vi "Search in 1D Array.vi"(2 "Task in":refnum<class "Task.lvclass">, 3 "Task Array":refnum<class "Task.lvclass">[](array[class])) -> (0 "index of element":i32, 1 "Task":refnum<class "Task.lvclass">)   [LabVIEW 2017, in "Task Interface.lvlib" / "Task.lvclass"]
uses:
  Task.lvclass
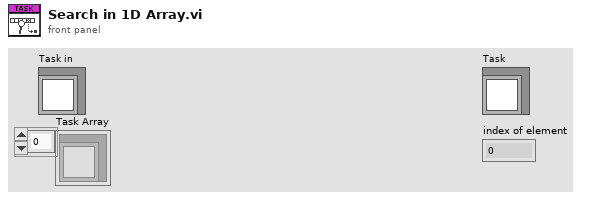
[diagram p1: front panel]
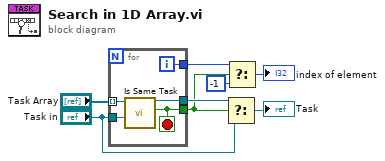
[diagram p0: block diagram]
diagram:
  n1 = for {
    tunnel: "Task Array" -> [w10] mode=indexing
    tunnel: "Task in" -> [w9]
    tunnel: [w12] -> w2
    tunnel: [w11] -> w8
    tunnel: [w10] -> w3
    i -> [w11]
    stop <- w12 stop-if-true
    n2 = call "Is Same Task.vi"("Task in 2"=w9, "Task in"=w10) -> ("Same Task?"=w12:bool)  [unwired: 9 in]
  }
  n3 = Select(t=w3, s=w2, f="Task in") -> (s? t:f=→"Task":refnum<class "Task.lvclass">)
  n4 = Select(t=w8, s=w2, f=-1) -> (s? t:f=→"index of element":i32)
